vi "PSU_initialize.vi"(9 "Current":dbl format="%.2f", 10 "Voltage":dbl format="%.2f", 11 "VISA resource name":refnum<visa-resource-name>="COM5") -> (3 "VISA resource name out":refnum<visa-resource-name>)   [LabVIEW 2023]
uses:
  <vilib>/Instr/_visa.llb/VISA Configure Serial Port (Instr).vi
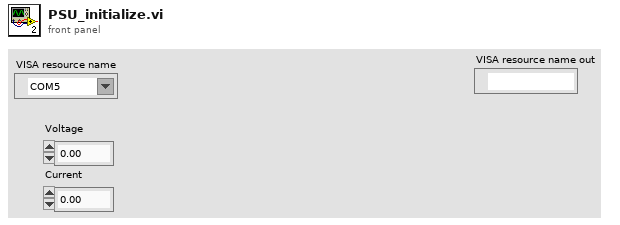
[diagram p1: front panel]
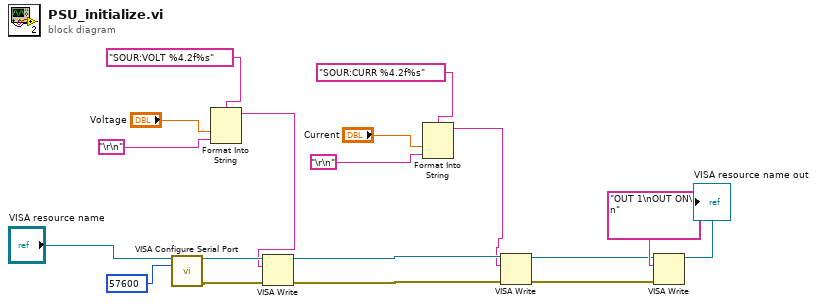
[diagram p0: block diagram]
diagram:
  n1 = call-poly "VISA Configure Serial Port"("VISA resource name"="VISA resource name", "baud rate (9600)"=u32 57600) -> ("VISA resource name out"=w15:refnum<visa-resource-name>, "error out"=w14:errorcluster)  [unwired: 12 in]
  n2 = Format Into String(format string="SOUR:VOLT %4.2f%s", "Voltage", "\r\n") -> (resulting string=w10:string)  [unwired: 2 in, 1 out]
  n3 = VISA Write(VISA resource name=w15, write buffer=w10, error in (no error)=w14) -> (VISA resource name out=w9:refnum<visa-resource-name>, error out=w8:errorcluster)  [unwired: 1 out]
  n4 = Format Into String(format string="SOUR:CURR %4.2f%s", "Current", "\r\n") -> (resulting string=w4:string)  [unwired: 2 in, 1 out]
  n5 = VISA Write(VISA resource name=w9, write buffer=w4, error in (no error)=w8) -> (VISA resource name out=w3:refnum<visa-resource-name>, error out=w2:errorcluster)  [unwired: 1 out]
  n6 = VISA Write(VISA resource name=w3, write buffer="OUT 1\nOUT ON\n", error in (no error)=w2) -> (VISA resource name out=→"VISA resource name out":refnum<visa-resource-name>)  [unwired: 2 out]
